vi "TRIGER.vi"(0 "Camera Handle":u32, 1 "Exposure (sec)":dbl format="%.3f", 2 "Number of frams":u32, 3 "Trigger Edge":u32, 7 "ReadOut Mode":u16(ring)=1 items=["Full Frame"=1, "Kinetics"=10], 11 "error out":errorcluster, 12 "Acquire / Focus Flag":u32, 13 "Timing Mode":u32) -> (4 "Camera Handle":u32, 6 "INI Flag":bool, 8 "String":string, 15 "error out":errorcluster)   [LabVIEW 2015]
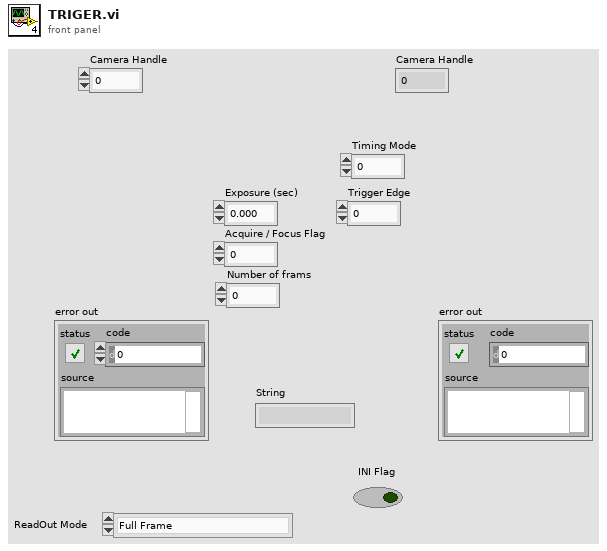
[diagram p1: front panel]
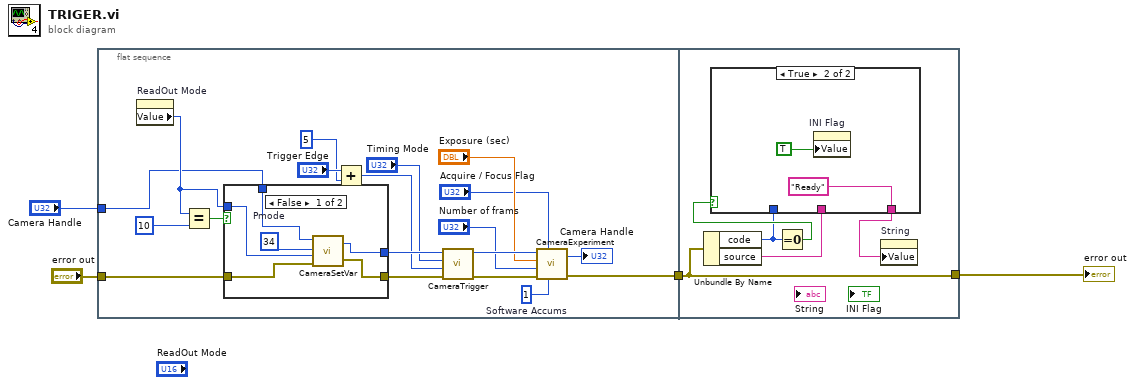
[diagram p0: block diagram]
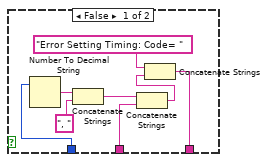
[diagram p3: hidden frame]
diagram:
  n1 = flat-sequence {
    tunnel: [w20] -> w4
    tunnel: "error out" -> [w17]
    tunnel: "Camera Handle" -> [w13]
    tunnel: w4 -> [w36]
    tunnel: [w36] -> w2
    frame #0 {
      w23 = 1  # Software Accums
      n2 = property on="ReadOut Mode" class="Ring (strict)"() -> ("Value"=w14:u16)  [unwired: 2 in, 2 out]
      n3 = Equal?(x=w14, y=10) -> (x = y?=w16:bool)
      n4 = case shown="False" w16 {
        tunnel: [w28 w31] -> w19
        tunnel: [w27 w30] -> w18
        tunnel: w17 -> [w26 w31]
        tunnel: w14 -> [w24 _]
        tunnel: w13 -> [w25 w30]
        frame False {
          w29 = 34  # Pmode
          n5 = call <userlib>:"CameraSetVar.vi"("error in"=w26, "Value"=w24, "Parameter ID"=w29, "Camera Handle"=w25) -> ("error out"=w28:errorcluster, "CameraHandle"=w27:u32)
        }
        frame True {
        }
      }
      n6 = Add(x="Trigger Edge", y=u32 5) -> (x+y=w6:u32)
      n7 = call <userlib>:"CameraTrigger.vi"("error in"=w19, "Trigger Edge"=w6, "Timing Mode"="Timing Mode", "Camera Handle"=w18) -> ("error out"=w21:errorcluster, "Camera Handle"=w22:u32)
      n8 = call <userlib>:"CameraExperiment.vi"("Number of Accumulations"=w23, "Acquire / Focus Flag"="Acquire / Focus Flag", "error in"=w21, "Number of Images"="Number of frams", "Exposure (sec)"="Exposure (sec)", "Camera Handle"=w22) -> ("error out"=w20:errorcluster, "Camera Handle"=→"Camera Handle":u32)
    }
    frame #1 {
      n9 = Unbundle By Name(w36) -> ("code"=w33:i32, "source"=w34:string)
      n10 = Equal To 0?(x=w33) -> (x = 0?=w35:bool)
      n11 = case shown="True" w35 {
        tunnel: [w37 "Ready"] -> w32
        tunnel: w34 -> [w38 _]
        tunnel: w33 -> [w43 _]
        frame False {
          n12 = Number To Decimal String(number=w43) -> (decimal integer string=w42:string)  [unwired: 1 in]
          n13 = Concatenate Strings(w42, ", ") -> (w39:string)
          n14 = Concatenate Strings(w39, w38) -> (w40:string)
          n15 = Concatenate Strings("Error Setting Timing: Code= ", w40) -> (w37:string)
        }
        frame True {
          n16 = property on="INI Flag" class="Bool (strict)"("Value"=TRUE) -> ()  [unwired: 2 in, 2 out]
        }
      }
      n17 = property on="String" class="Str"("Value"=w32) -> ()  [unwired: 2 in, 2 out]
    }
  }
  "error out" <- w2
